vi "06.3 Create an Execution Log File.vi"() -> ()   [LabVIEW 2019]
uses:
  Support Files/02.4 DAQmx Configuration Cluster.ctl
  Support Files/03.2 States.ctl
  Support Files/03.2 State Machine Data.ctl
  <vilib>/DAQmx/read.llb/DAQmx Read (Analog 2D DBL NChan NSamp).vi
  <vilib>/DAQmx/write.llb/DAQmx Write (Analog DBL 1Chan 1Samp).vi
  <vilib>/DAQmx/create/channels.llb/DAQmx Create Channel (AI-Voltage-Basic).vi
  <vilib>/DAQmx/configure/timing.llb/DAQmx Timing (Sample Clock).vi
  <vilib>/DAQmx/miscellaneous.llb/DAQmx Fill In Error Info.vi
  <vilib>/Utility/file.llb/Write Delimited Spreadsheet (string).vi
  <vilib>/Utility/file.llb/Write Delimited Spreadsheet (DBL).vi
  <vilib>/DAQmx/create/channels.llb/DAQmx Create Channel (AO-Voltage-Basic).vi
panel:
  in  "DAQmx Configuration Cluster":T1={"Desired Sample Rate (Hz)"=-1.0, "sample mode"=10178, "Minimum value"=-1.0, "Maximum value"=-1.0, "Physical Channel"="", "units"=10143, "thermocouple type"=10072, "Samples per Channel"=0} {"thermocouple type" items=["J"=10072, "K"=10073, "N"=10077, "R"=10082, "S"=10085, "T"=10086, "B"=10047, "E"=10055]; "units" items=["Deg C"=10143, "Deg F"=10144, "Kelvins"=10325, "Deg R"=10145, "From Custom Scale"=10065]; "sample mode" items=["Finite Samples"=10178, "Continuous Samples"=10123, "Hardware Timed Single Point"=12522]}
  in  "Threshold (RMS)":dbl
  in  "Generate Stimulus":bool
  in  "Stop":bool
  in  "Clear":bool
  in  "Acquire":bool
  out "Graph":dbl[][](graph)
  out "Thershold Exceeded?":bool
  out "RMS Result per Channel":dbl[](array[numeric])
  # "ANALYSIS"
  # "EVENTS"
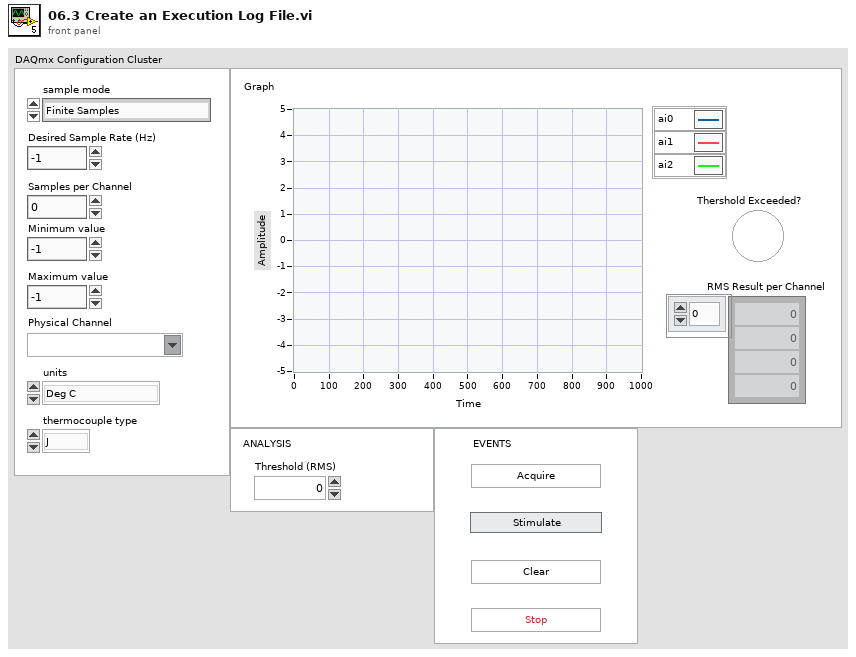
[diagram p1: front panel]
types:
  T1 = typedef "02.4 DAQmx Configuration Cluster.ctl" = cluster{"Desired Sample Rate (Hz)":dbl, "sample mode":i32, "Minimum value":dbl, "Maximum value":dbl, "Physical Channel":tag, "units":i32, "thermocouple type":i32, "Samples per Channel":i32}
  T2 = enum16{"open", "replace", "create", "open or create", "replace or create", "replace or create with confirmation"}
  T3 = typedef "03.2 State Machine Data.ctl" = cluster{"Acquisition Data":dbl[][], "Stimulus?":bool}
  T4 = typedef "03.2 States.ctl" = enum16{"Initialize", "Update UI", "Update Stimulus", "Wait for event", "Acquire", "Analyze", "Log", "Clear", "Shutdown"}
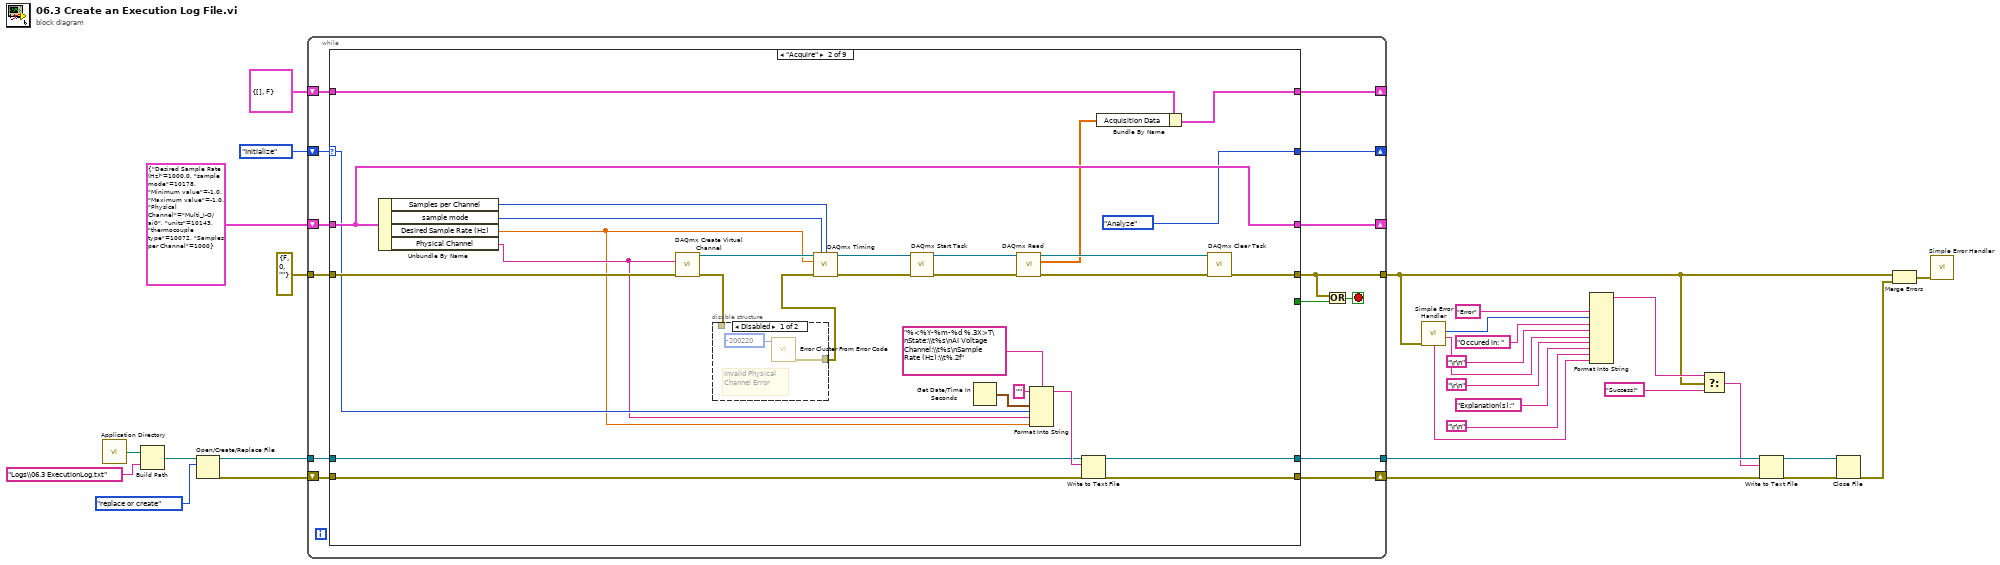
[diagram p0: block diagram]
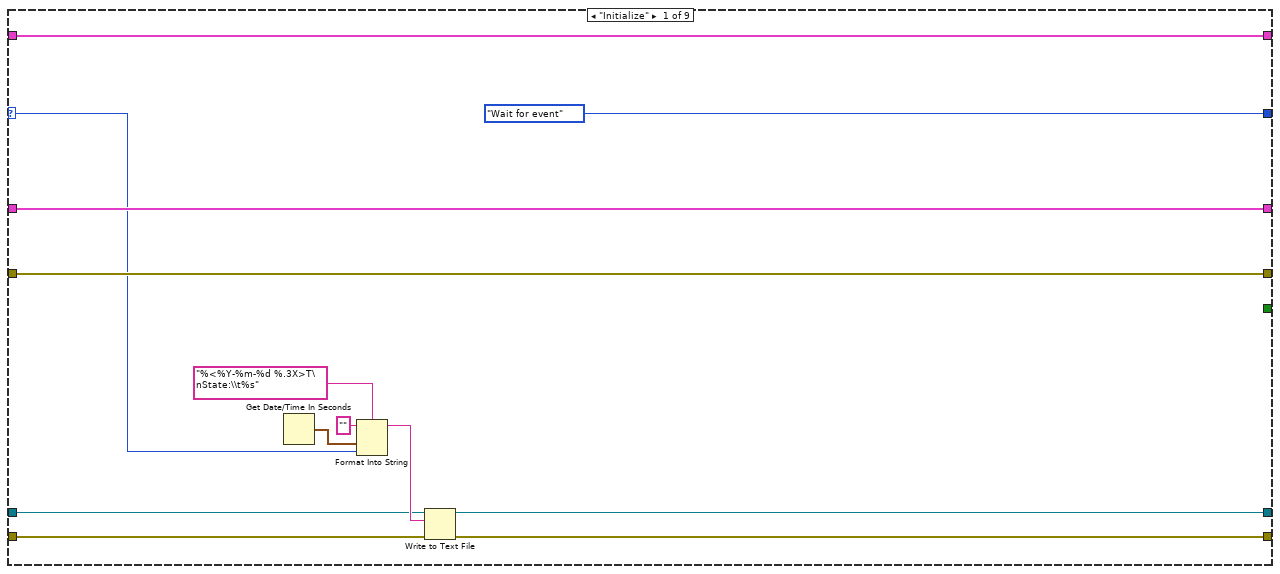
[diagram p2: hidden frame]
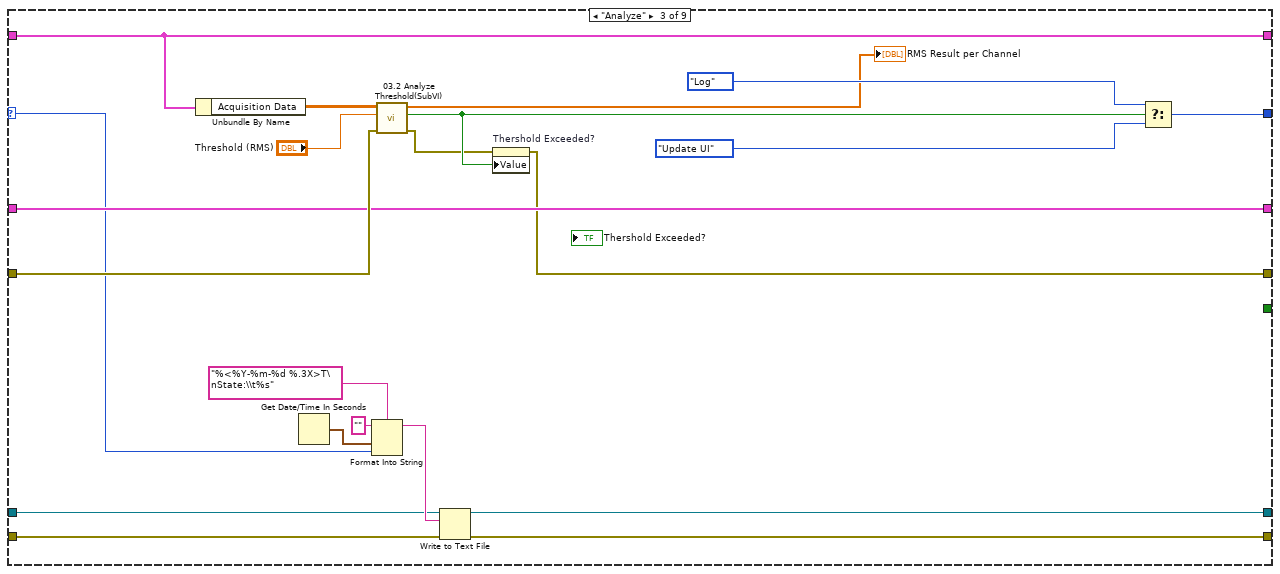
[diagram p4: hidden frame]
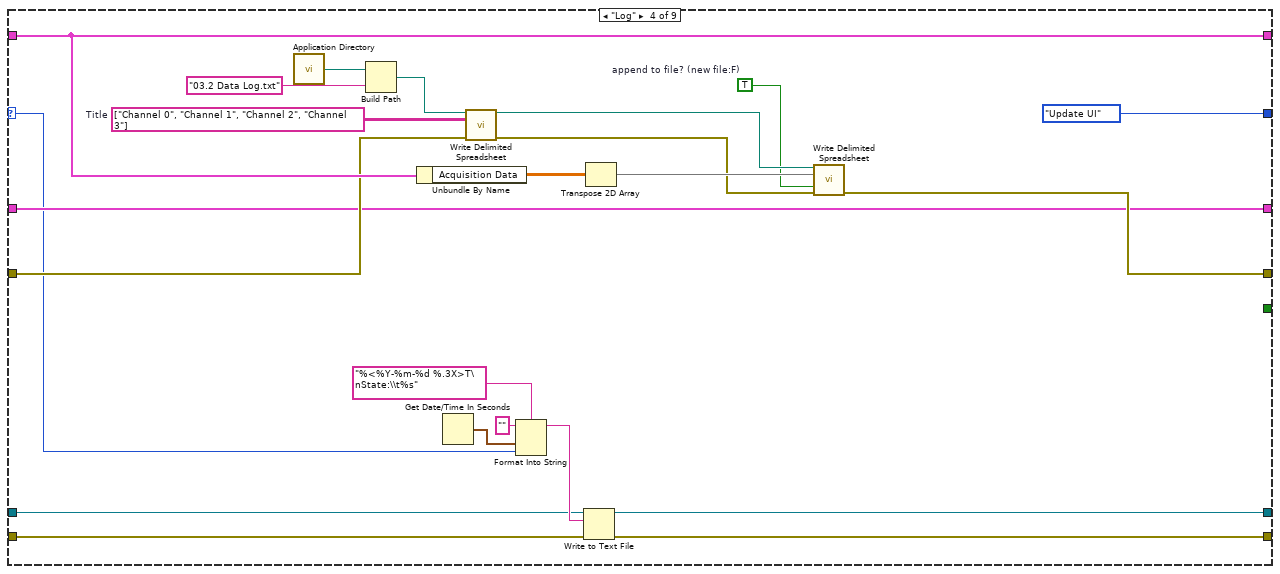
[diagram p5: hidden frame]
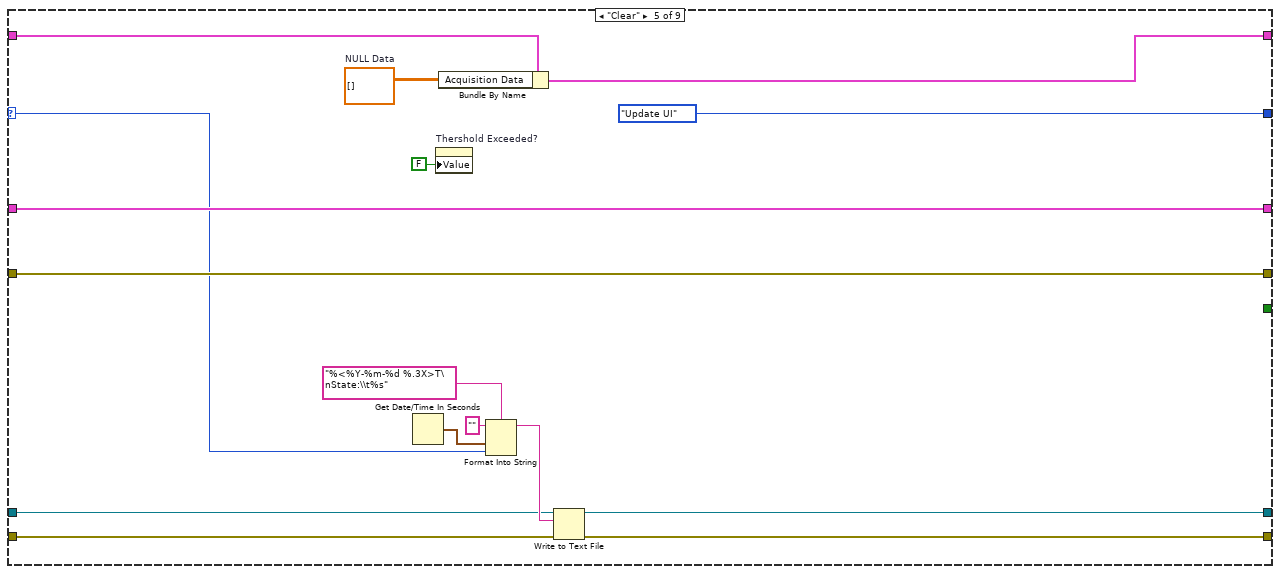
[diagram p6: hidden frame]
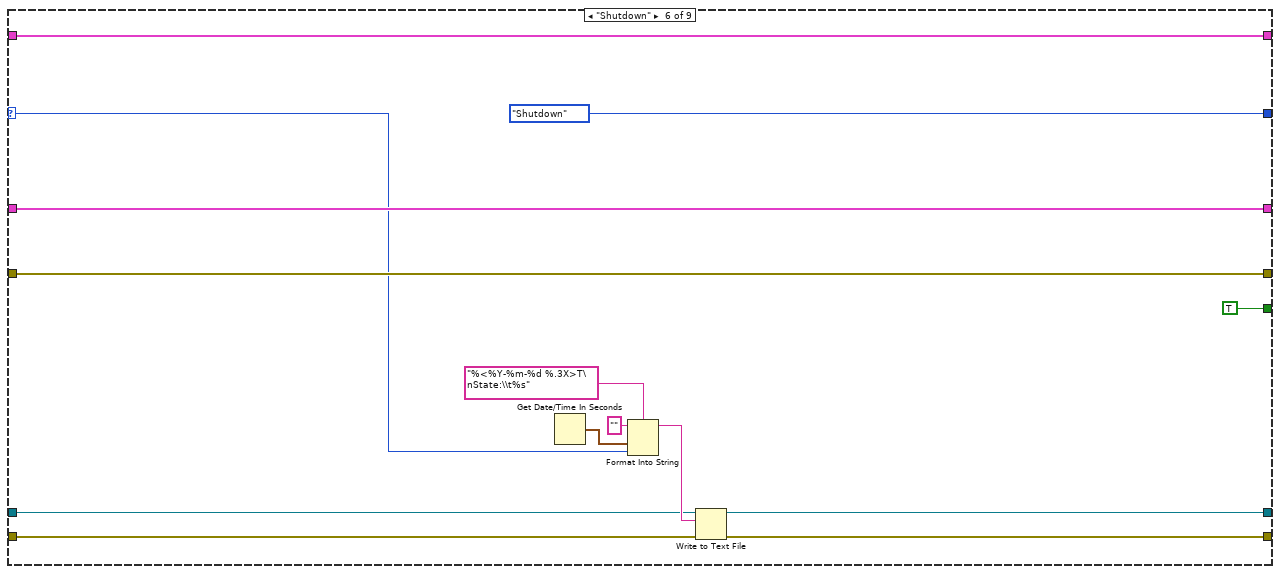
[diagram p7: hidden frame]
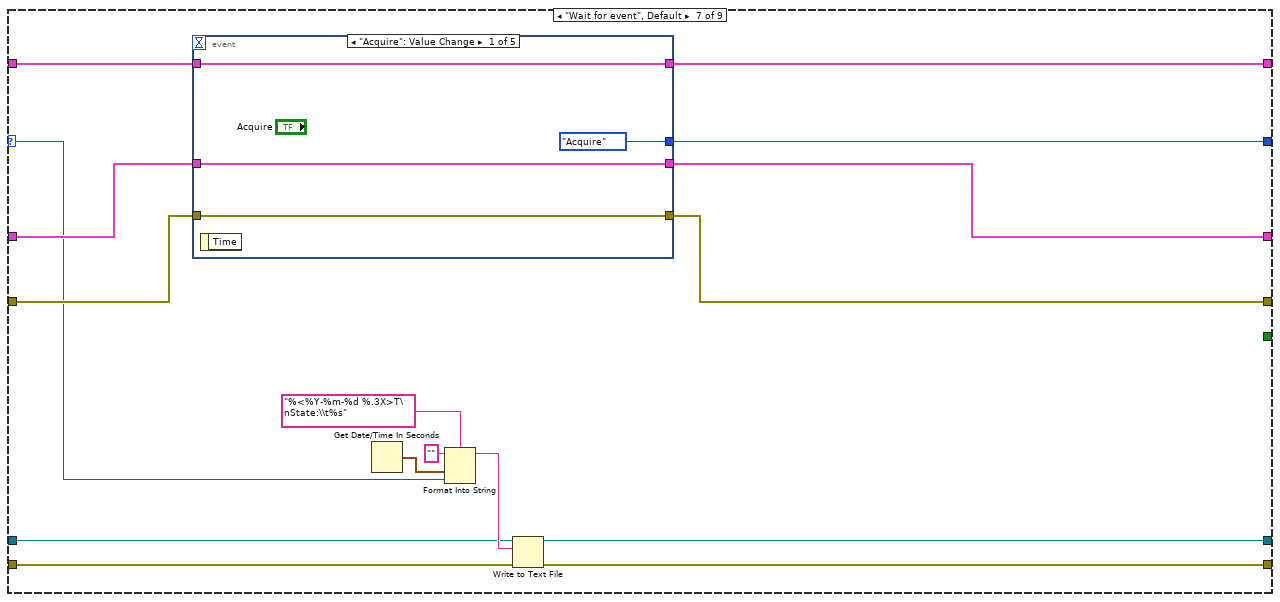
[diagram p8: hidden frame]
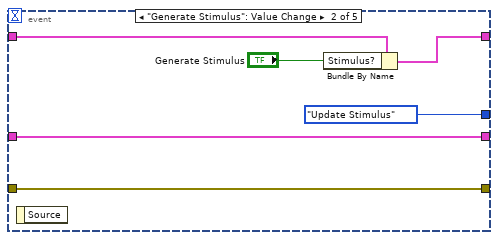
[diagram p9: hidden frame]
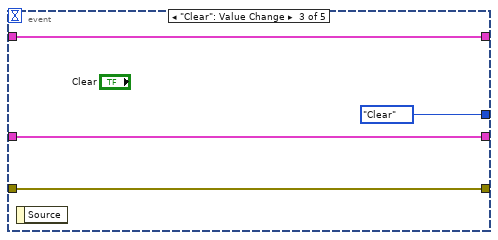
[diagram p10: hidden frame]
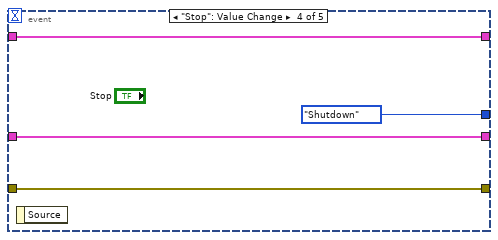
[diagram p11: hidden frame]
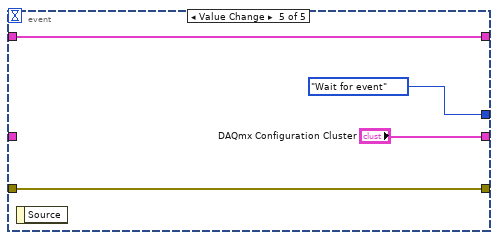
[diagram p12: hidden frame]
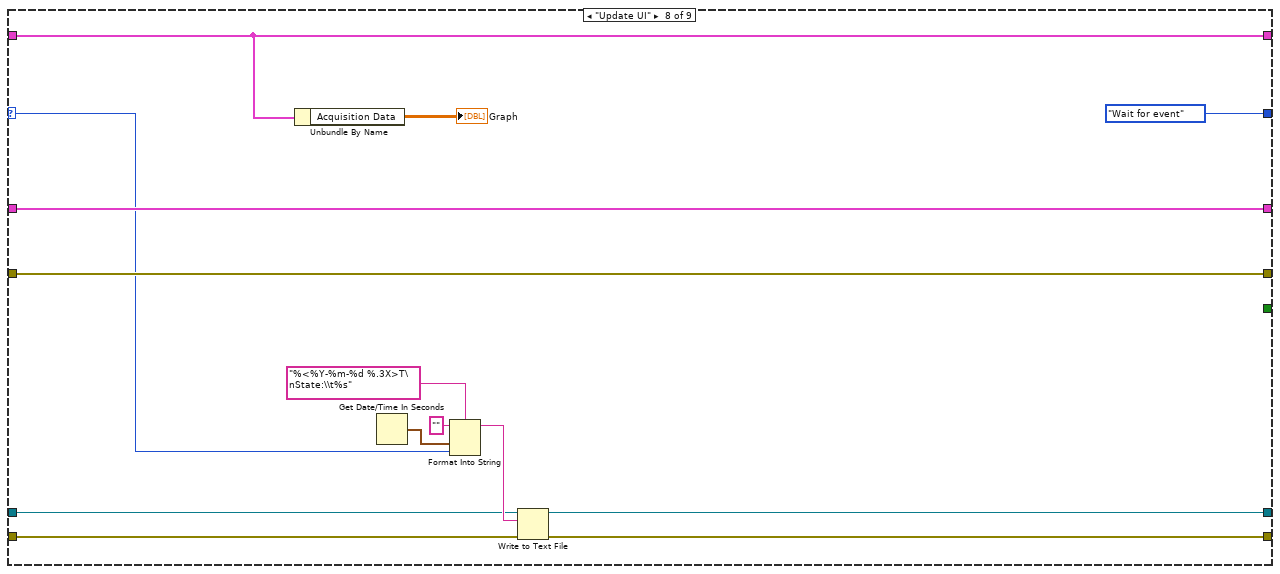
[diagram p13: hidden frame]
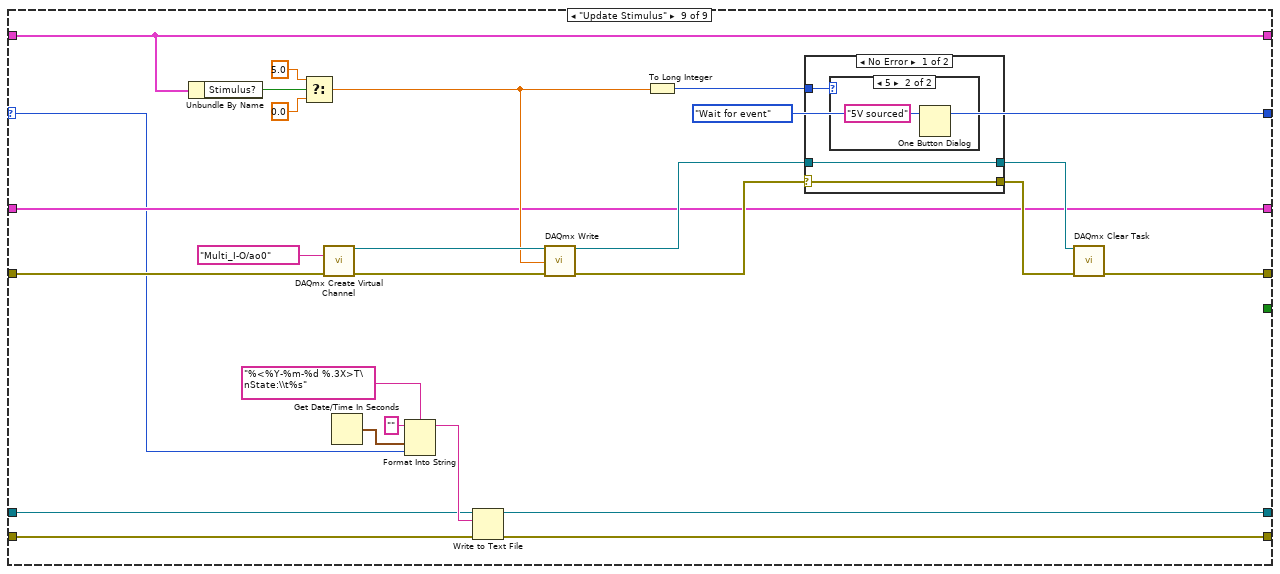
[diagram p14: hidden frame]
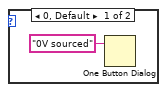
[diagram p15: hidden frame]
diagram:
  n1 = call <vilib>:"Application Directory.vi"() -> ("Application Directory"=w21:path)
  n2 = Build Path(base path=w21, name or relative path="Logs\\06.3 ExecutionLog.txt") -> (appended path=w22:path)
  n3 = Open/Create/Replace File(file path (use dialog)=w22, operation (0:open)=T2."replace or create") -> (refnum out=w23:refnum<file>, error out=w24:errorcluster)  [unwired: 4 in, 1 out]
  n4 = while {
    shift-right: [w42] -> _
    shift-left: 03.2_States."Initialize" ("State") -> [w43]
    tunnel: errorcluster {"status"=FALSE, "code"=0, "source"=""} ("error constant") -> [w41]
    tunnel: [w39] -> w3
    shift-right: [w38] -> _
    shift-left: T3 {"Acquisition Data"=[], "Stimulus?"=FALSE} -> [w37]
    shift-right: [w34] -> _
    shift-left: T1 {"Desired Sample Rate (Hz)"=1000.0, "sample mode"=10178, "Minimum value"=-1.0, "Maximum value"=-1.0, "Physical Channel"="Multi_I-O/ai0", "units"=10143, "thermocouple type"=10072, "Samples per Channel"=1000} ("DAQmx Configuration Cluster") -> [w35]
    shift-right: [w31] -> w8
    shift-left: w24 -> [w32]
    tunnel: w23 -> [w33]
    tunnel: [w30] -> w7
    stop <- w40 stop-if-true
    n5 = case shown="\"Acquire\"" w43 {
      selector: w43 -> [w46 w69 w89 w110 w133 w149 w163 w201 w215]
      tunnel: [03.2_States."Wait for event" ("State") 03.2_States."Analyze" ("State") w108 03.2_States."Update UI" ("State") 03.2_States."Update UI" ("State") 03.2_States."Shutdown" ("State") w178 03.2_States."Wait for event" ("State") 03.2_States."Wait for event" ("State")] -> w42
      tunnel: [w55 w82 w98 w130 w144 w160 w177 w212 w229] -> w39
      tunnel: w41 -> [w55 w83 w105 w120 w144 w160 w176 w212 w240]
      tunnel: [w56 w76 w104 w128 w147 w161 w175 w214 w226] -> w38
      tunnel: w37 -> [w56 w78 w104 w128 w148 w161 w174 w214 w226]
      tunnel: [_ _ _ _ _ TRUE _ _ _] -> w36
      tunnel: w35 -> [w53 w79 w100 w119 w143 w158 w173 w210 w225]
      tunnel: [w53 w79 w100 w119 w143 w158 w172 w210 w225] -> w34
      tunnel: w33 -> [w48 w64 w93 w114 w137 w153 w167 w205 w219]
      tunnel: w32 -> [w47 w60 w92 w113 w136 w152 w166 w204 w218]
      tunnel: [w44 w63 w91 w112 w135 w151 w164 w203 w217] -> w30
      tunnel: [w45 w62 w90 w111 w134 w150 w165 w202 w216] -> w31
      frame "Initialize" {
        n6 = Get Date/Time In Seconds() -> (seconds since 1Jan1904=w52:timestamp)
        n7 = Format Into String "Format Into String"(format string="%<%Y-%m-%d %.3X>T\nState:\\t%s", initial string="", w52, w46) -> (resulting string=w51:string)  [unwired: 1 in, 1 out]
        n8 = Write to Text File(file (use dialog)=w48, text=w51, error in=w47) -> (refnum out=w44:refnum<file>, error out=w45:errorcluster)  [unwired: 1 in, 1 out]
      }
      frame "Acquire" {
        n9 = Unbundle By Name(w79) -> ("Samples per Channel"=w66:i32, "sample mode"=w84:i32, "Desired Sample Rate (Hz)"=w67:dbl, "Physical Channel"=w68:tag)
        n10 = call-poly <vilib>:"DAQmx Create Virtual Channel.vi"("physical channels"=w68, "error in"=w83) -> ("task out"=w85:refnum<k21>, "error out"=w58:errorcluster)  [unwired: 12 in]
        n11 = disable-structure shown="Disabled" {
          disable-tunnel: [w86 w88] -> w57
          disable-tunnel: w58 -> [_ w88]
          frame Disabled {
            # "Invalid Physical Channel Error"
            n12 = call <vilib>:"Error Cluster From Error Code.vi"("error code (0)"=-200220 ("specific error code to clear (0: all)")) -> ("error out"=w86:errorcluster)  [unwired: 8 in]
          }
          frame Enabled {
          }
        }
        n13 = call-poly <vilib>:"DAQmx Timing.vi"("task/channels in"=w85, "sample mode"=w84, "samples per channel"=w66, "rate"=w67, "error in"=w57) -> ("task out"=w71:refnum<k21>, "error out"=w72:errorcluster)  [unwired: 9 in]
        n14 = call <vilib>:"DAQmx Start Task.vi"("task/channels in"=w71, "error in"=w72) -> ("task out"=w73:refnum<k21>, "error out"=w74:errorcluster)  [unwired: 12 in]
        n15 = Get Date/Time In Seconds() -> (seconds since 1Jan1904=w70:timestamp)
        n16 = call-poly <vilib>:"DAQmx Read.vi"("task/channels in"=w73, "error in"=w74) -> ("task out"=w80:refnum<k21>, "data"=w77:dbl[][], "error out"=w81:errorcluster)  [unwired: 11 in]
        n17 = Format Into String "Format Into String"(format string="%<%Y-%m-%d %.3X>T\nState:\\t%s\nAI Voltage Channel:\\t%s\nSample Rate (Hz):\\t%.2f", initial string="", w70, w69, w68, w67) -> (resulting string=w65:string)  [unwired: 1 in, 1 out]
        n18 = Write to Text File(file (use dialog)=w64, text=w65, error in=w60) -> (refnum out=w63:refnum<file>, error out=w62:errorcluster)  [unwired: 1 in, 1 out]
        n19 = Bundle By Name(cluster=w78, "Acquisition Data"=w77) -> (w76:T3)
        n20 = call <vilib>:"DAQmx Clear Task.vi"("task in"=w80, "error in"=w81) -> ("error out"=w82:errorcluster)  [unwired: 13 in]
      }
      frame "Analyze" {
        n21 = Unbundle By Name(w104) -> ("Acquisition Data"=w109:dbl[][])
        n22 = Get Date/Time In Seconds() -> (seconds since 1Jan1904=w97:timestamp)
        n23 = Format Into String "Format Into String"(format string="%<%Y-%m-%d %.3X>T\nState:\\t%s", initial string="", w97, w89) -> (resulting string=w96:string)  [unwired: 1 in, 1 out]
        n24 = call "03.2 Analyze Threshold(SubVI).vi"("Error In"=w105, "Threshold (RMS)"="Threshold (RMS)", "Data"=w109) -> ("Error Out"=w99:errorcluster, "Threshold exceeded?"=w101:bool, "RMS Results per Channel"=→"RMS Result per Channel":dbl[])  [unwired: 6 in]
        n25 = Write to Text File(file (use dialog)=w93, text=w96, error in=w92) -> (refnum out=w91:refnum<file>, error out=w90:errorcluster)  [unwired: 1 in, 1 out]
        n26 = property on="Thershold Exceeded?" class="Bool (strict)"(error in=w99, "Value"=w101) -> (error out=w98:errorcluster)  [unwired: 1 in, 1 out]
        n27 = Select(t=03.2_States."Log" ("State"), s=w101, f=03.2_States."Update UI" ("State")) -> (s? t:f=w108:T4)
      }
      frame "Log" {
        w122 = string[][] [["Channel 0", "Channel 1", "Channel 2", "Channel 3"]]  # Title
        w124 = TRUE  # append to file? (new file:F)
        n28 = call <vilib>:"Application Directory.vi"() -> ("Application Directory"=w132:path)
        n29 = Build Path(base path=w132, name or relative path="03.2 Data Log.txt") -> (appended path=w123:path)
        n30 = Unbundle By Name(w128) -> ("Acquisition Data"=w127:dbl[][])
        n31 = Get Date/Time In Seconds() -> (seconds since 1Jan1904=w118:timestamp)
        n32 = call-poly <vilib>:"Write Delimited Spreadsheet.vi"("file path (dialog if empty)"=w123, "2D data"=w122, "error in (no error)"=w120) -> ("new file path (Not A Path if cancelled)"=w125:path, "error out"=w121:errorcluster)  [unwired: 11 in]
        n33 = Format Into String "Format Into String"(format string="%<%Y-%m-%d %.3X>T\nState:\\t%s", initial string="", w118, w110) -> (resulting string=w117:string)  [unwired: 1 in, 1 out]
        n34 = Write to Text File(file (use dialog)=w114, text=w117, error in=w113) -> (refnum out=w112:refnum<file>, error out=w111:errorcluster)  [unwired: 1 in, 1 out]
        n35 = Transpose 2D Array(2D array=w127) -> (transposed array=w126:dbl[][])
        n36 = call-poly <vilib>:"Write Delimited Spreadsheet.vi"("file path (dialog if empty)"=w125, "2D data"=w126, "append to file? (new file:F)"=w124, "error in (no error)"=w121) -> ("error out"=w130:errorcluster)  [unwired: 10 in, 1 out]
      }
      frame "Clear" {
        w146 = dbl[][] []  # NULL Data
        n37 = Get Date/Time In Seconds() -> (seconds since 1Jan1904=w141:timestamp)
        n38 = property on="Thershold Exceeded?" class="Bool (strict)"("Value"=FALSE ("Thershold Exceeded?")) -> ()  [unwired: 2 in, 2 out]
        n39 = Bundle By Name(cluster=w148, "Acquisition Data"=w146) -> (w147:T3)
        n40 = Format Into String "Format Into String"(format string="%<%Y-%m-%d %.3X>T\nState:\\t%s", initial string="", w141, w133) -> (resulting string=w140:string)  [unwired: 1 in, 1 out]
        n41 = Write to Text File(file (use dialog)=w137, text=w140, error in=w136) -> (refnum out=w135:refnum<file>, error out=w134:errorcluster)  [unwired: 1 in, 1 out]
      }
      frame "Shutdown" {
        n42 = Get Date/Time In Seconds() -> (seconds since 1Jan1904=w157:timestamp)
        n43 = Format Into String "Format Into String"(format string="%<%Y-%m-%d %.3X>T\nState:\\t%s", initial string="", w157, w149) -> (resulting string=w156:string)  [unwired: 1 in, 1 out]
        n44 = Write to Text File(file (use dialog)=w153, text=w156, error in=w152) -> (refnum out=w151:refnum<file>, error out=w150:errorcluster)  [unwired: 1 in, 1 out]
      }
      frame "Wait for event", Default {
        n45 = event shown="[0] \"Acquire\": Value Change" {
          selector: _ -> [_ _ _ _ _]
          dyn-events: _ -> [_ _ _ _ _]
          timeout: _ -> [_ _ _ _ _]
          tunnel: [03.2_States."Acquire" ("State") 03.2_States."Update Stimulus" ("State") 03.2_States."Clear" ("State") 03.2_States."Shutdown" ("State") 03.2_States."Wait for event" ("State")] -> w178
          tunnel: [w181 w184 w190 w195 w197] -> w177
          tunnel: w176 -> [w181 w184 w190 w195 w197]
          tunnel: [w180 w186 w192 w194 w199] -> w175
          tunnel: w174 -> [w180 w188 w192 w194 w199]
          tunnel: w173 -> [w179 w183 w189 w193 _]
          tunnel: [w179 w183 w189 w193 "DAQmx Configuration Cluster"] -> w172
          event "Acquire": Value Change {
            n46 = event-data() -> ()  [unwired: 1 in, 1 out]
          }
          event "Generate Stimulus": Value Change {
            n47 = event-data() -> ()  [unwired: 1 in, 1 out]
            n48 = Bundle By Name(cluster=w188, "Stimulus?"="Generate Stimulus") -> (w186:T3)
          }
          event "Clear": Value Change {
            n49 = event-data() -> ()  [unwired: 1 in, 1 out]
          }
          event "Stop": Value Change {
            n50 = event-data() -> ()  [unwired: 1 in, 1 out]
          }
          event Value Change {
            n51 = event-data() -> ()  [unwired: 1 in, 1 out]
          }
        }
        n52 = Get Date/Time In Seconds() -> (seconds since 1Jan1904=w171:timestamp)
        n53 = Format Into String "Format Into String"(format string="%<%Y-%m-%d %.3X>T\nState:\\t%s", initial string="", w171, w163) -> (resulting string=w170:string)  [unwired: 1 in, 1 out]
        n54 = Write to Text File(file (use dialog)=w167, text=w170, error in=w166) -> (refnum out=w164:refnum<file>, error out=w165:errorcluster)  [unwired: 1 in, 1 out]
      }
      frame "Update UI" {
        n55 = Unbundle By Name(w214) -> ("Acquisition Data"=→"Graph":dbl[][])
        n56 = Get Date/Time In Seconds() -> (seconds since 1Jan1904=w208:timestamp)
        n57 = Format Into String "Format Into String"(format string="%<%Y-%m-%d %.3X>T\nState:\\t%s", initial string="", w208, w201) -> (resulting string=w209:string)  [unwired: 1 in, 1 out]
        n58 = Write to Text File(file (use dialog)=w205, text=w209, error in=w204) -> (refnum out=w203:refnum<file>, error out=w202:errorcluster)  [unwired: 1 in, 1 out]
      }
      frame "Update Stimulus" {
        n59 = Unbundle By Name(w226) -> ("Stimulus?"=w237:bool)
        n60 = Select(t=5.0, s=w237, f=0.0) -> (s? t:f=w234:dbl)
        n61 = call-poly <vilib>:"DAQmx Create Virtual Channel.vi"("physical channels"=tag "Multi_I-O/ao0", "error in"=w240) -> ("task out"=w238:refnum<k21>, "error out"=w239:errorcluster)  [unwired: 12 in]
        n62 = Get Date/Time In Seconds() -> (seconds since 1Jan1904=w223:timestamp)
        n63 = Format Into String "Format Into String"(format string="%<%Y-%m-%d %.3X>T\nState:\\t%s", initial string="", w223, w215) -> (resulting string=w222:string)  [unwired: 1 in, 1 out]
        n64 = Write to Text File(file (use dialog)=w219, text=w222, error in=w218) -> (refnum out=w217:refnum<file>, error out=w216:errorcluster)  [unwired: 1 in, 1 out]
        n65 = call-poly <vilib>:"DAQmx Write.vi"("task/channels in"=w238, "data"=w234, "error in"=w239) -> ("task out"=w232:refnum<k21>, "error out"=w233:errorcluster)  [unwired: 10 in, 1 out]
        n66 = To Long Integer(number=w234) -> (32bit integer=w227:i32)
        n67 = case shown="No Error" w233 {
          selector: w233 -> [w243 w246]
          tunnel: w232 -> [w242 w247]
          tunnel: [w243 w246] -> w231
          tunnel: [w242 w247] -> w230
          tunnel: w227 -> [w241 _]
          frame No Error {
            n68 = case shown="5" w241 {
              frame 0, Default {
                n69 = One Button Dialog(message="0V sourced") -> ()  [unwired: 1 in, 1 out]
              }
              frame 5 {
                n70 = One Button Dialog(message="5V sourced") -> ()  [unwired: 1 in, 1 out]
              }
            }
          }
          frame Error {
          }
        }
        n71 = call <vilib>:"DAQmx Clear Task.vi"("task in"=w230, "error in"=w231) -> ("error out"=w229:errorcluster)  [unwired: 13 in]
      }
    }
    n72 = Or(x=w39, y=w36) -> (x .or. y?=w40:bool)
  }
  n73 = call <vilib>:"Simple Error Handler.vi"("error in (no error)"=w3) -> ("code out"=w18:i32, "source out"=w15:string, "message"=w11:string)  [unwired: 4 in, 2 out]
  n74 = Format Into String "Format Into String"("Error", w18, "Occured in: ", "\r\n", w15, "\r\n", "Explanation(s):", "\r\n", w11) -> (resulting string=w10:string)  [unwired: 3 in, 1 out]
  n75 = Select(t=w10, s=w3, f="Success!") -> (s? t:f=w6:string)
  n76 = Write to Text File(file (use dialog)=w7, text=w6, error in=w8) -> (refnum out=w5:refnum<file>, error out=w4:errorcluster)  [unwired: 1 in, 1 out]
  n77 = Close File(refnum=w5, error in=w4) -> (error out=w2:errorcluster)  [unwired: 1 out]
  n78 = Merge Errors(w3, w2) -> (w1:errorcluster)
  n79 = call <vilib>:"Simple Error Handler.vi"("error in (no error)"=w1) -> ()  [unwired: 4 in, 5 out]
